vi "Test Database.vi"() -> ()   [LabVIEW 2017]
uses:
  <vilib>/addons/database/Connection.llb/DB Tools Open Connec (Path).vi
  <vilib>/addons/database/NI_Database_API.lvlib
panel:
  out "error out":errorcluster
  in  "connection information":path
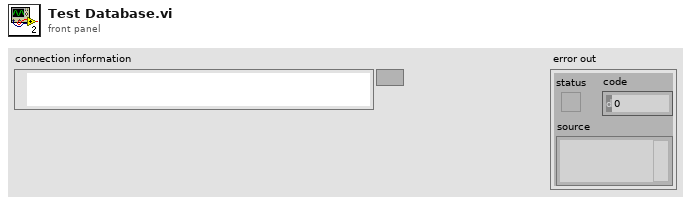
[diagram p1: front panel]
types:
  T1 = typedef "NI_Database_API.lvlib/Conn ObjectReference.ctl" = refnum<k1>
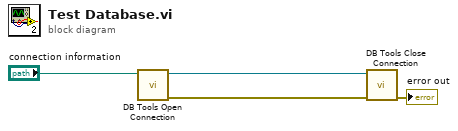
[diagram p0: block diagram]
diagram:
  n1 = call-poly <vilib>:"DB Tools Open Connection.vi"("connection information"="connection information") -> ("error out"=w2:errorcluster, "connection reference"=w3:T1)  [unwired: 7 in]
  n2 = call <vilib>:"DB Tools Close Connection.vi"("error in (no error)"=w2, "connection reference"=w3) -> ("error out"=→"error out":errorcluster)  [unwired: 5 in]
